vi "RPC Method ni_measurements_v1_MeasurementService_Measure Logic.vi"(8 "error in":errorcluster, 11 "gRPCid in":T1) -> (0 "error out":errorcluster)   [LabVIEW 2020, in "LineRegulation.lvlib" / "MeasurementService.lvclass"]
uses:
  MeasurementService.lvclass
  <vilib>/gRPC/LabVIEW gRPC Library/Server API/typeDefs/grpcId.ctl
  Measurement Configuration.ctl
  <vilib>/gRPC/LabVIEW gRPC Library/Server API/typeDefs/gRPC Status Code.ctl
  0672971e-e56b-41b4-b8c2-ef1eaad3a7f7.vi
  d8da19cd-d6a4-4014-b7d8-b1c6013a3d24.vi
  <vilib>/gRPC/LabVIEW gRPC Library/Server API/Server/Get Server DLL Path.vi
  LineRegulation.lvlib
  <vilib>/gRPC/LabVIEW gRPC Library/gprc-lvsupport-release.lvlib
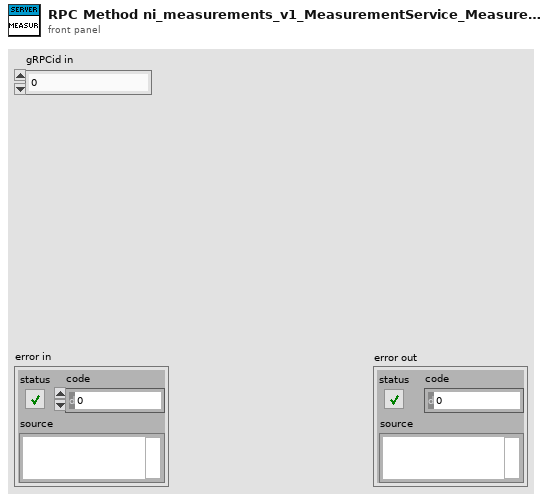
[diagram p1: front panel]
types:
  T1 = typedef "gprc-lvsupport-release.lvlib/grpcId.ctl" = u64
  T2 = typedef "LineRegulation.lvlib/Measurement Configuration.ctl" = cluster{"Load Current in A":dbl, "Nominal Output Voltage in V":dbl, "Start":dbl, "Stop":dbl, "Step":dbl, "Input SMU":string, "Load SMU":string, "Input DMM":string, "Load DMM":string}
  T3 = typedef "LineRegulation.lvlib/ni_measurements_v1_MeasureRequest.ctl" = cluster{"configuration_parameters":T4}
  T4 = typedef "LineRegulation.lvlib/google_protobuf_Any.ctl" = cluster{"type_url":string, "value":u8[]}
  T5 = typedef "LineRegulation.lvlib/Measurement Results.ctl" = cluster{"Line Regulation (%/V)":dbl, "Line Regulation (%)":dbl, "Output Voltage in V":dbl[], "Test Results.Input Voltage in V":dbl[]}
  T6 = typedef "gprc-lvsupport-release.lvlib/gRPC Status Code.ctl" = enum16{"OK", "CANCELLED", "UNKNOWN", "INVALID_ARGUMENT", "DEADLINE_EXCEEDED", "NOT_FOUND", "ALREADY_EXISTS", "PERMISSION_DENIED", "RESOURCE_EXHAUSTED", "FAILED_PRECONDITION", "ABORTED", "OUT_OF_RANGE", "UNIMPLEMENTED", "INTERNAL", "UNAVAILABLE", "DATA_LOSS", "UNAUTHENTICATED"}
  T7 = typedef "gprc-lvsupport-release.lvlib/Any.ctl" = cluster{"Type Url":string, "Bytes":u8[]}
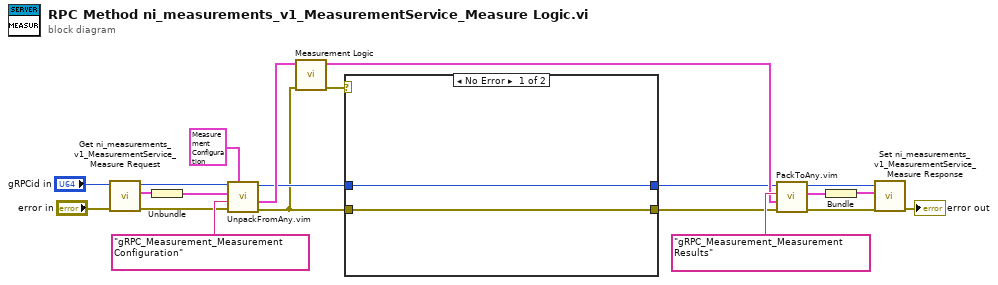
[diagram p0: block diagram]
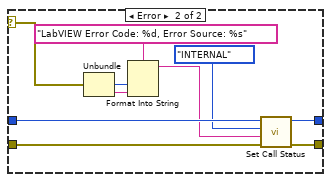
[diagram p2: hidden frame]
diagram:
  n1 = call "Get ni_measurements_v1_MeasurementService_Measure Request.vi"("error in (no error)"="error in", "gRPCid in"="gRPCid in") -> ("error out"=w14:errorcluster, "Message Data"=w15:T3, "gRPCid out"=w13:T1)  [unwired: 7 in]
  n2 = Unbundle(w15) -> ("configuration_parameters"=w21:T4)
  n3 = call "UnpackFromAny.vim"("Data Type"=T2 {"Load Current in A"=0.005, "Nominal Output Voltage in V"=3.3, "Start"=4.0, "Stop"=6.0, "Step"=0.1, "Input SMU"="", "Load SMU"="", "Input DMM"="", "Load DMM"=""} ("Measurement Configuration"), "error in (no error)"=w14, "Message Type"="gRPC_Measurement_Measurement Configuration", "Any"=w21, "gRPCid in"=w13) -> ("error out"=w5:errorcluster, "Unpacked Value"=w17:T2, "gRPCid"=w7:u64)  [unwired: 4 in]
  n4 = call "Measurement Logic.vi"("error in"=w5, "Measurement Configuration"=w17) -> ("error out"=w8:errorcluster, "Measurement Results"=w18:T5)  [unwired: 8 in]
  n5 = case shown="No Error" w8 {
    selector: w8 -> [_ w33]
    tunnel: w7 -> [w23 w32]
    tunnel: [w23 w31] -> w6
    tunnel: w5 -> [w22 w29]
    tunnel: [w22 w30] -> w4
    frame No Error {
    }
    frame Error {
      n6 = Unbundle(w33) -> ("code"=w27:i32, "source"=w26:string)  [unwired: 1 out]
      n7 = Format Into String(format string="LabVIEW Error Code: %d, Error Source: %s", w27, w26) -> (resulting string=w24:string)  [unwired: 2 in, 1 out]
      n8 = call <vilib>:"Set Call Status.vi"("error in (no error)"=w29, "Details"=w24, "Status Code"=gRPC_Status_Code."INTERNAL", "gRCP ID"=w32) -> ("error out"=w30:errorcluster, "gRCP ID Out"=w31:T1)  [unwired: 6 in]
    }
  }
  n9 = call "PackToAny.vim"("error in (no error)"=w4, "Data To Pack"=w18, "Message Type"="gRPC_Measurement_Measurement Results", "gRPCid in"=w6) -> ("error out"=w9:errorcluster, "Any"=w11:T7, "gRPCid"=w12:u64)  [unwired: 5 in]
  n10 = Bundle("Any"=w11) -> (w10:cluster{"Any":T7})  [unwired: 1 in]
  n11 = call "Set ni_measurements_v1_MeasurementService_Measure Response.vi"("error in (no error)"=w9, "Message Data"=w10, "gRPCid in"=w12) -> ("error out"=→"error out":errorcluster)  [unwired: 8 in]
